vi "XBox-Globals.vi"() -> ()   [LabVIEW 2015]
uses:
  XBox-Button Event.ctl
  XBox-Events Ref.ctl
panel:
  out "Connected?":bool
  out "XBox Event Ref":T1
  out "XBox Events":T2
  out "Stop?":bool
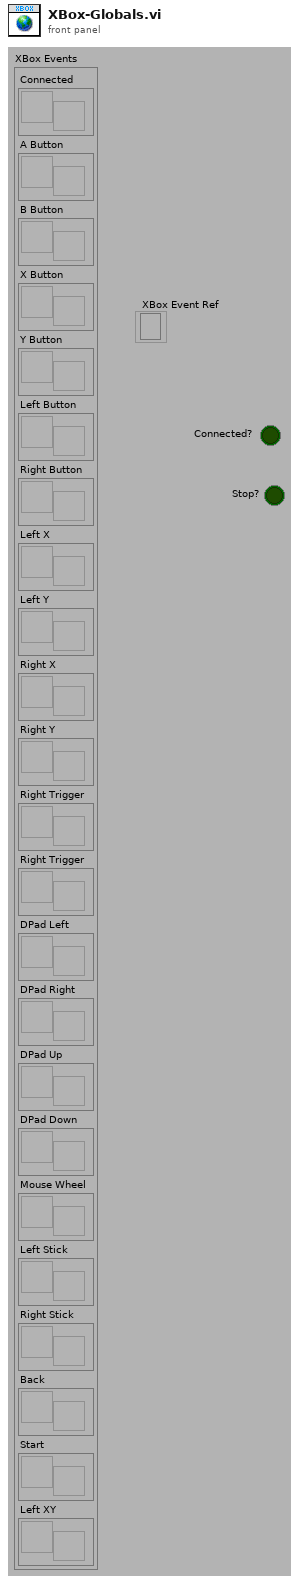
[diagram p1: front panel]
types:
  T1 = typedef "XBox-Events Ref.ctl" = refnum<event-registration>
  T2 = cluster{"Connected":refnum<user-event>, "A Button":refnum<user-event>, "B Button":refnum<user-event>, "X Button":refnum<user-event>, "Y Button":refnum<user-event>, "Left Button":refnum<user-event>, "Right Button":refnum<user-event>, "Left X":refnum<user-event>, "Left Y":refnum<user-event>, "Right X":refnum<user-event>, "Right Y":refnum<user-event>, "Right Trigger":refnum<user-event>, "Right Trigger":refnum<user-event>, "DPad Left":refnum<user-event>, "DPad Right":refnum<user-event>, "DPad Up":refnum<user-event>, "DPad Down":refnum<user-event>, "Mouse Wheel":refnum<user-event>, "Left Stick":refnum<user-event>, "Right Stick":refnum<user-event>, "Back":refnum<user-event>, "Start":refnum<user-event>, "Left XY":refnum<user-event>}
diagram:
